vi "Read Teller Metadata.vi"(11 "Base Teller in":refnum<class "Base Teller.lvclass">) -> (2 "Teller Metadata":refnum<class "Teller Metadata.lvclass">)   [LabVIEW 2020, in "jettl.lvlib" / "Base Teller.lvlib" / "Base Teller.lvclass"]
uses:
  Base Teller.lvclass
  Teller Metadata/Teller Metadata.lvclass
  Base Teller.lvclass/Base Teller.ctl
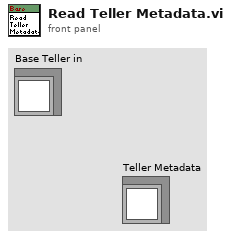
[diagram p1: front panel]
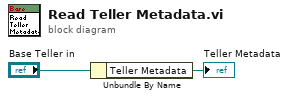
[diagram p0: block diagram]
diagram:
  n1 = Unbundle By Name("Base Teller in") -> ("Teller Metadata"=→"Teller Metadata":refnum<class "Teller Metadata.lvclass">)
